vi "Save VI ConPane Image__ogtk.vi"(5 "Image Depth (256)":i32=256, 7 "Image Format":enum32{"PNG", "JPEG", "GIF"}(ring)=enum."GIF", 8 "error in (no error)":errorcluster, 10 "Image File Path":path, 11 "VI Path":path) -> (0 "error out":errorcluster)   [LabVIEW 2020]
doc: "Save an image to file of a VI's Connector Pane."
uses:
  <userlib>/_OpenG.lib/file/file.llb/Strip Path - Traditional__ogtk.vi
  <userlib>/_OpenG.lib/file/file.llb/Build Path - Traditional__ogtk.vi
panel:
  # "Save VI ConPane Image.vi\n\nSave an image to file of a VI's Connector Pane.\n\nPlease visit http://www.OpenG.org to learn about the\nOpen Source LabVIEW software movement.\n\nNOTICE -- YOU MUST LEAVE THIS NOTICE IN PLACE.  PER THE TERMS OF THE LICENSE BELOW, YOU MAY SUBLICENSE THIS SOFTWARE \nIN ANY WAY THAT DOES NOT CONFLICT WITH THIS LICENSE.\n\n### BSD License (http://www.opensource.org/licenses/bsd-license.php) Begin ###\n \nCopyright (c) 2002, Jim Kring <jim@jimkring.com>\n\nAll rights reserved.\n\nRedistribution and use in source and binary forms, with or without modification, are permitted provided that the following conditions are met:\n\n    * Redistributions of source code must retain the above copyright notice, this list of conditions and the following disclaimer.\n    * Redistributions in binary form must reproduce the above copyright notice, this list of conditions and the following disclaimer in the \n       documentation and/or other materials provided with the distribution.\n    * Neither the name of SciWare, James Kring, Inc., nor the names of its contributors may be used to endorse or promote products derived \n       from this software without specific prior written permission.\n\nTHIS SOFTWARE IS PROVIDED BY THE COPYRIGHT HOLDERS AND CONTRIBUTORS \"AS IS\" AND ANY EXPRESS OR IMPLIED WARRANTIES, \nINCLUDING, BUT NOT LIMITED TO, THE IMPLIED WARRANTIES OF MERCHANTABILITY AND FITNESS FOR A PARTICULAR PURPOSE ARE \nDISCLAIMED. IN NO EVENT SHALL THE COPYRIGHT OWNER OR CONTRIBUTORS BE LIABLE FOR ANY DIRECT, INDIRECT, INCIDENTAL,\n SPECIAL, EXEMPLARY, OR CONSEQUENTIAL DAMAGES (INCLUDING, BUT NOT LIMITED TO, PROCUREMENT OF SUBSTITUTE GOODS OR \nSERVICES; LOSS OF USE, DATA, OR PROFITS; OR BUSINESS INTERRUPTION) HOWEVER CAUSED AND ON ANY THEORY OF LIABILITY, \nWHETHER IN CONTRACT, STRICT LIABILITY, OR TORT (INCLUDING NEGLIGENCE OR OTHERWISE) ARISING IN ANY WAY OUT OF THE USE \nOF THIS SOFTWARE, EVEN IF ADVISED OF THE POSSIBILITY OF SUCH DAMAGE.\n\n### BSD License End ###"
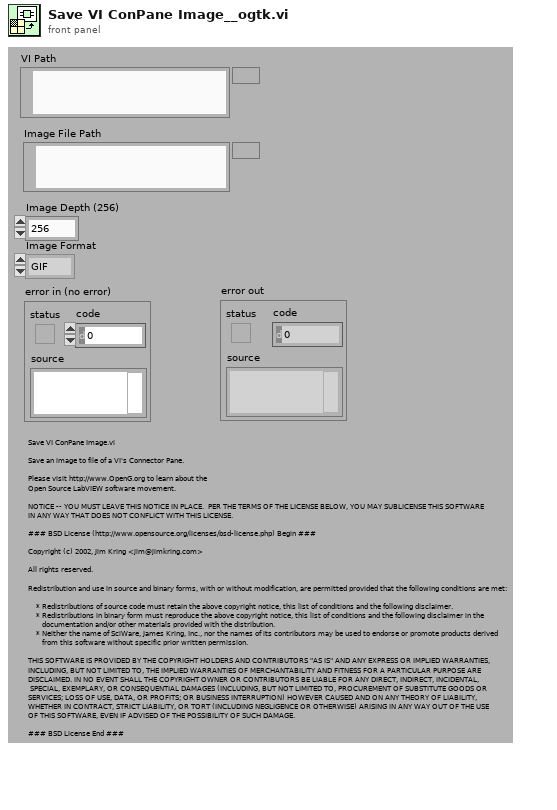
[diagram p1: front panel]
types:
  T1 = enum32{"Custom", "Standard", "Using Panel", "Using SubVI", "Complete"}
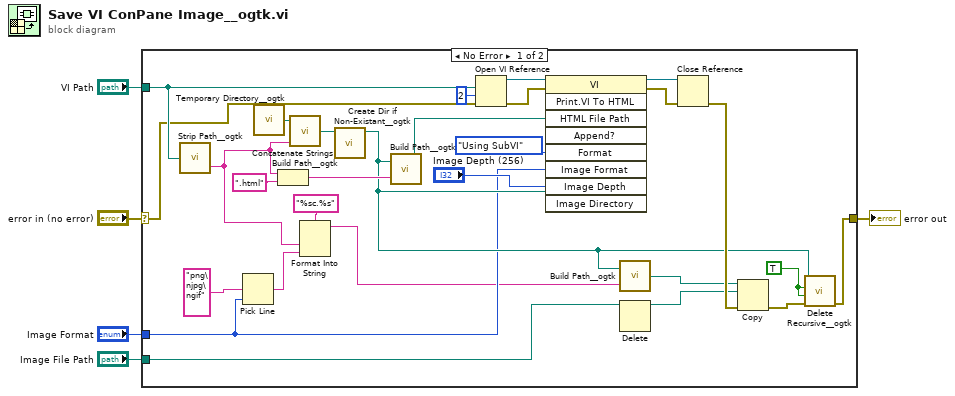
[diagram p0: block diagram]
diagram:
  n1 = case shown="No Error" "error in (no error)" {
    selector: "error in (no error)" -> [w8 w34]
    tunnel: "VI Path" -> [w20 _]
    tunnel: [w19 w34] -> w4
    tunnel: "Image File Path" -> [w16 _]
    tunnel: "Image Format" -> [w11 _]
    frame No Error {
      w18 = TRUE ("Recursive? (FALSE)")
      n2 = call-poly <userlib>:"Strip Path__ogtk.vi"("path"=w20) -> ("name"=w7:string)  [unwired: 1 out]
      n3 = Pick Line(multi-line string="png\njpg\ngif", line index=w11) -> (output string=w12:string)  [unwired: 1 in]
      n4 = call <userlib>:"Temporary Directory__ogtk.vi"() -> ("Temporary Directory (+ Relative)"=w26:path)  [unwired: 1 in]
      n5 = Concatenate Strings(w7, ".html" ("Substring")) -> (w28:string)
      n6 = call-poly <userlib>:"Build Path__ogtk.vi"("name or relative path"=w7, "base path"=w26) -> ("appended path"=w30:path)
      n7 = Format Into String(format string="%sc.%s" ("Format String"), w7, w12) -> (resulting string=w9:string)  [unwired: 2 in, 1 out]
      n8 = call <userlib>:"Create Dir if Non-Existant__ogtk.vi"("Directory Path"=w30) -> ("dup Directory Path"=w14:path)  [unwired: 8 in, 2 out]
      n9 = call-poly <userlib>:"Build Path__ogtk.vi"("name or relative path"=w28, "base path"=w14) -> ("appended path"=w29:path)
      n10 = Open VI Reference(vi path=w20, options=2, error in (no error)=w8) -> (vi reference=w24:refnum<vi>, error out=w32:errorcluster)  [unwired: 3 in]
      n11 = invoke class="VI" method="Print.VI To HTML"(reference=w24, error in=w32, "HTML File Path"=w29, "Format"=T1."Using SubVI", "Image Format"=w11, "Image Depth"="Image Depth (256)", "Image Directory"=w14) -> (reference out=w31:refnum<vi>, error out=w33:errorcluster)  [unwired: 2 in, 7 out]
      n12 = call-poly <userlib>:"Build Path__ogtk.vi"("name or relative path"=w9, "base path"=w14) -> ("appended path"=w17:path)
      n13 = Delete(path (use dialog)=w16) -> (deleted path=w15:path)  [unwired: 4 in, 2 out]
      n14 = Close Reference(reference=w31, error in (no error)=w33) -> (error out=w22:errorcluster)
      n15 = Copy(8:w22, 10:w15, 11:w17) -> (0:w21:errorcluster)  [unwired: 2 in, 2 out]
      n16 = call <userlib>:"Delete Recursive__ogtk.vi"("error in (no error)"=w21, "Ignore Read-Only? (FALSE)"=w18, "Recursive? (FALSE)"=w18, "Path"=w14) -> ("error out"=w19:errorcluster)  [unwired: 6 in, 1 out]
    }
    frame Error {
    }
  }
  "error out" <- w4
